vi "Get Build Steps core.vi"(8 "error in (no error)":errorcluster, 9 "Preview?":bool, 10 "Build Configuration":string, 11 "Caraya Item in":refnum<class "Caraya Item.lvclass">) -> (0 "error out":errorcluster, 2 "Build Steps":refnum<class "Build Step.lvclass">[](array[class]))   [LabVIEW 2019, in "Caraya Library.lvlib" / "Caraya Item.lvclass"]
uses:
  Caraya Item.lvclass
  libs/Solution.lvlibp/Solution/Build Item/Build Step.lvclass
  Caraya Item.lvclass/Caraya Item.ctl
  Run Tests Step/Run Tests Step.lvclass
  C:/Users/pasca/source/repos/mgi-solution-explorer-extensions/libs/Solution.lvlibp/Solution/Build Item/Build Step.lvclass
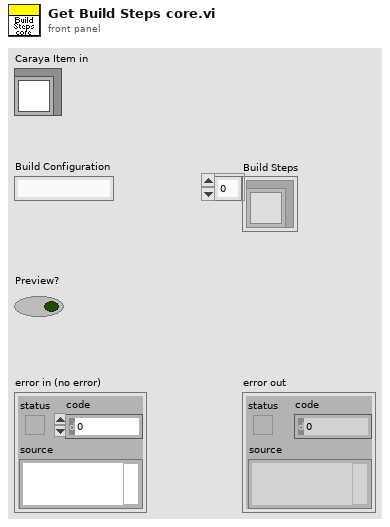
[diagram p1: front panel]
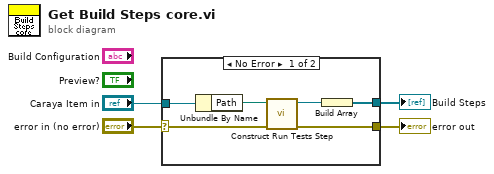
[diagram p0: block diagram]
diagram:
  n1 = case shown="No Error" "error in (no error)" {
    selector: "error in (no error)" -> [w10 w11]
    tunnel: [w9 w11] -> w3
    tunnel: "Caraya Item in" -> [w8 _]
    tunnel: [w7 _] -> w1
    frame No Error {
      n2 = Unbundle By Name(w8) -> ("Path"=w6:path)
      n3 = call "Construct Run Tests Step.vi"("error in (no error)"=w10, "Path"=w6) -> ("error out"=w9:errorcluster, "Run Tests Step"=w5:refnum<class "Run Tests Step.lvclass">)  [unwired: 8 in]
      n4 = Build Array(w5) -> (w7:refnum<class "Run Tests Step.lvclass">[])
    }
    frame Error {
    }
  }
  "error out" <- w3
  "Build Steps" <- w1
